vi "List Policy Versions.vi"(8 "error in (no error)":errorcluster, 10 "Name":string, 11 "IoT Session in":refnum<class "IoT Session.lvclass">) -> (0 "error out":errorcluster, 2 "Versions":T1[](array[typedef]) {"Creation Date" format="%#_12g"}, 3 "IoT Session out":refnum<class "IoT Session.lvclass">)   [LabVIEW 2015, in "NI_AWS_IoT.lvlib" / "IoT Session.lvclass"]
uses:
  IoT Session.lvclass
  Policy Version.ctl
  Core/HTTP Request/Request Options.ctl
  Core/HTTP Request/Name Value Pair.ctl
  Core/HTTP Request/Region handling.ctl
  Core/HTTP Request/URL formatting.ctl
  Core/HTTP Request/HTTP Request.lvclass
  JSON Parsing/NI_JSON Parsing.lvlib
  NI_AWS_IoT.lvlib
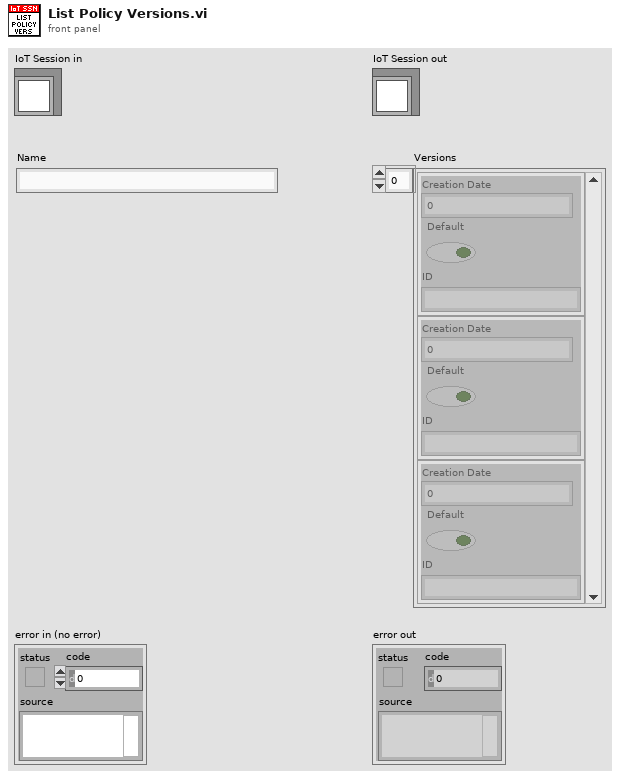
[diagram p1: front panel]
types:
  T1 = typedef "NI_AWS_IoT.lvlib/Policy Version.ctl" = cluster{"Creation Date":dbl, "Default":bool, "ID":string}
  T2 = typedef "NI_AWS_Core.lvlib/HTTP Request.lvclass/Name Value Pair.ctl" = cluster{"name":string, "value":string}
  T3 = typedef "NI_AWS_Core.lvlib/HTTP Request.lvclass/Request Options.ctl" = cluster{"request headers":T2[], "request parameters":T2[], "request body":string, "region handling":T4, "URL formatting":T5}
  T4 = typedef "NI_AWS_Core.lvlib/HTTP Request.lvclass/Region handling.ctl" = enum16{"use region everywhere", "use region (authentication only)", "use region (URL only)", "ignore region everwhere"}
  T5 = typedef "NI_AWS_Core.lvlib/HTTP Request.lvclass/URL formatting.ctl" = enum16{"region-", "region."}
  T6 = typedef "NI_AWS_Core.lvlib/HTTP Request.lvclass/Response.ctl" = cluster{"Headers":string, "Body":string}
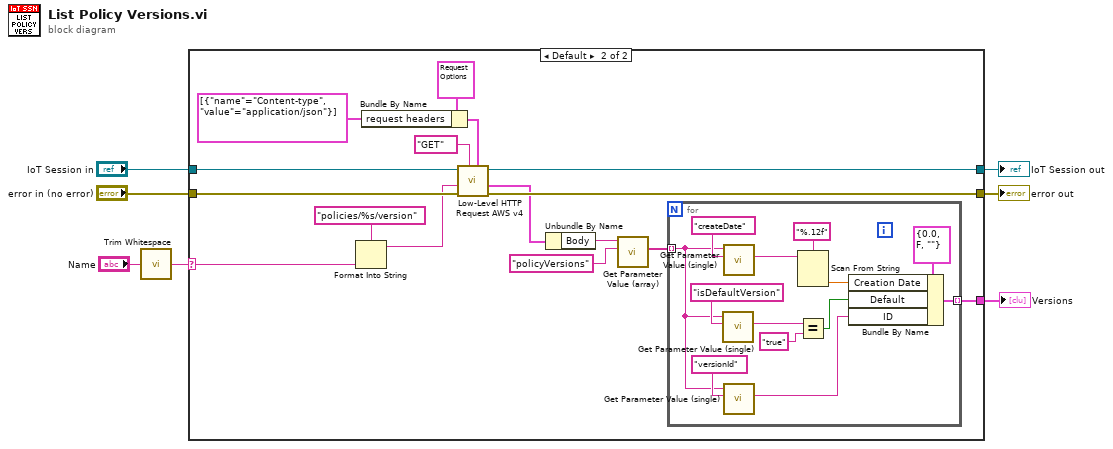
[diagram p0: block diagram]
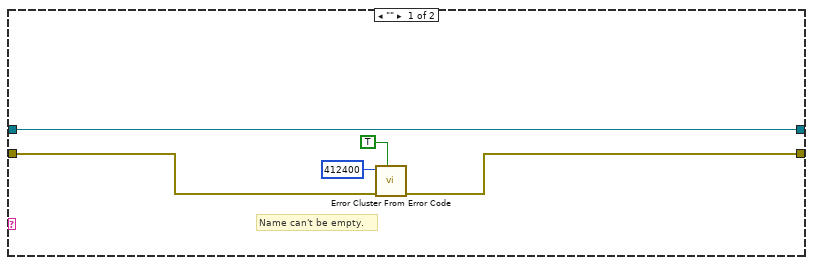
[diagram p2: hidden frame]
diagram:
  n1 = call <vilib>:"Trim Whitespace.vi"("string"="Name") -> ("trimmed string"=w2:string)  [unwired: 1 in]
  n2 = case shown="Default" w2 {
    selector: w2 -> [_ w14]
    tunnel: "error in (no error)" -> [w9 w28]
    tunnel: [w8 w27] -> w6
    tunnel: [w12 w26] -> w5
    tunnel: "IoT Session in" -> [w12 w25]
    tunnel: [_ w13] -> w1
    frame "" {
      # "Name can't be empty."
      n3 = call <vilib>:"Error Cluster From Error Code.vi"("show call chain? (False)"=TRUE, "error in (no error)"=w9, "error code (0)"=412400) -> ("error out"=w8:errorcluster)  [unwired: 6 in]
    }
    frame Default {
      n4 = Format Into String(format string="policies/%s/version" ("string"), w14) -> (resulting string=w15:string)  [unwired: 2 in, 1 out]
      n5 = Bundle By Name(cluster=T3 {"request headers"=[], "request parameters"=[], "request body"="", "region handling"=enum."use region everywhere", "URL formatting"=enum."region."} ("Request Options"), "request headers"=T2[] [{"name"="Content-type", "value"="application/json"}]) -> (w22:T3)
      n6 = call "Low-Level HTTP Request AWS v4.vi"("Request Options"=w22, "HTTP-Verb"="GET", "error in (no error)"=w28, "URL Suffix"=w15, "AWS Core in"=w25) -> ("error out"=w27:errorcluster, "Response"=w20:T6, "AWS Core out"=w26:refnum<class "IoT Session.lvclass">)  [unwired: 3 in, 1 out]
      n7 = Unbundle By Name(w20) -> ("Body"=w19:string)
      n8 = call "Get Parameter Value (array).vi"("Parameter Name"="policyVersions", "JSON"=w19) -> ("Parameter Values"=w17:string[])  [unwired: 7 in, 2 out]
      n9 = for {
        tunnel: w17 -> [w30] mode=indexing
        tunnel: [w39] -> w13 mode=indexing
        n10 = call "Get Parameter Value (single).vi"("Parameter Name"="isDefaultVersion", "JSON"=w30) -> ("Parameter Value"=w34:string)  [unwired: 6 in, 3 out]
        n11 = call "Get Parameter Value (single).vi"("Parameter Name"="createDate", "JSON"=w30) -> ("Parameter Value"=w37:string)  [unwired: 6 in, 3 out]
        n12 = call "Get Parameter Value (single).vi"("Parameter Name"="versionId", "JSON"=w30) -> ("Parameter Value"=w29:string)  [unwired: 6 in, 3 out]
        n13 = Scan From String(format string="%.12f", input string=w37) -> (output 1=w36:dbl)  [unwired: 3 in, 3 out]
        n14 = Equal?(x=w34, y="true") -> (x = y?=w33:bool)
        n15 = Bundle By Name(cluster=T1 {"Creation Date"=0.0, "Default"=FALSE, "ID"=""} ("Policy Version"), "Creation Date"=w36, "Default"=w33, "ID"=w29) -> (w39:T1)
      }
    }
  }
  "error out" <- w6
  "IoT Session out" <- w5
  "Versions" <- w1
